vi "GoToPosition.vi"(8 "error in (no error)":errorcluster, 10 "Position":dbl[](array[numeric]), 11 "Serial Controller in":refnum<class "Serial Controller.lvclass">) -> (0 "error out":errorcluster, 3 "Serial Controller out":refnum<class "Serial Controller.lvclass">)   [LabVIEW 2012, in "Serial Controller.lvclass"]
uses:
  Serial Controller.lvclass
  Serial Controller.lvclass/Serial Controller.ctl
panel:
  out "Moving":bool
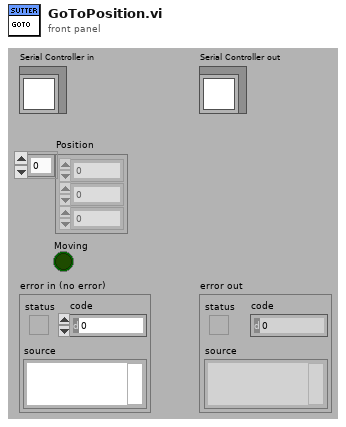
[diagram p1: front panel]
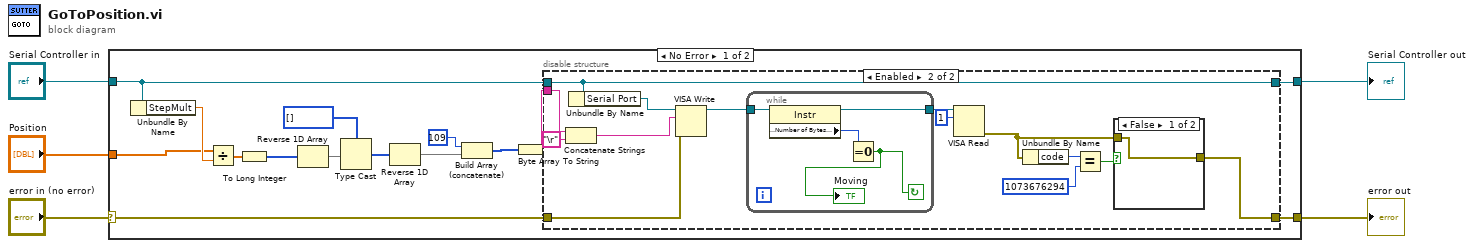
[diagram p0: block diagram]
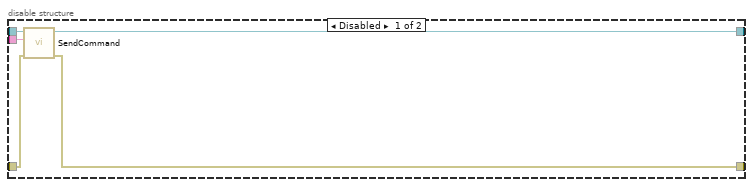
[diagram p2: hidden frame]
diagram:
  n1 = case shown="No Error" "error in (no error)" {
    selector: "error in (no error)" -> [w12 w46]
    tunnel: [w6 w46] -> w4
    tunnel: [w13 w45] -> w2
    tunnel: "Serial Controller in" -> [w14 w45]
    tunnel: "Position" -> [w15 _]
    frame No Error {
      n2 = Unbundle By Name(w14) -> ("StepMult"=w17:dbl)
      n3 = Divide(x=w15, y=w17) -> (x/y=w16:dbl[])
      n4 = To Long Integer(number=w16) -> (32bit integer=w8:i32[])
      n5 = Reverse 1D Array(array=w8) -> (reversed array=w11:i32[])
      n6 = Type Cast(type=u8[] [], x=w11) -> (*(type *) &x=w10:u8[])
      n7 = Reverse 1D Array(array=w10) -> (reversed array=w9:u8[])
      n8 = Build Array (concatenate)(u8 109, w9) -> (w18:u8[])
      n9 = Byte Array To String(unsigned byte array=w18) -> (string=w7:string)
      n10 = disable-structure shown="Enabled" {
        disable-tunnel: w14 -> [w25 w39]
        disable-tunnel: w7 -> [w24 w38]
        disable-tunnel: [w23 w39] -> w13
        disable-tunnel: w12 -> [w21 w34]
        disable-tunnel: [w22 w26] -> w6
        frame Disabled {
          n11 = call-dynamic "SendCommand.vi"("error in (no error)"=w21, "command"=w24, "Serial Controller in"=w25) -> ("error out"=w22:errorcluster, "Serial Controller out"=w23:refnum<class "Serial Controller.lvclass">)  [unwired: 6 in, 1 out]
        }
        frame Enabled {
          n12 = Concatenate Strings(w38, "\r" ("string")) -> (w35:string)
          n13 = Unbundle By Name(w39) -> ("Serial Port"=w36:refnum<visa-resource-name>)
          n14 = VISA Write(VISA resource name=w36, write buffer=w35, error in (no error)=w34) -> (VISA resource name out=w33:refnum<visa-resource-name>)  [unwired: 2 out]
          n15 = while {
            tunnel: w33 -> [w44]
            tunnel: [w42] -> w32
            stop <- w41 continue-if-true
            n16 = property class="Instr"(reference=w44) -> (reference out=w42:refnum<visa-resource-name>, "Serial Settings:Number of Bytes at Serial Port"=w43:u32)  [unwired: 1 in, 1 out]
            n17 = Equal To 0?(x=w43) -> (x = 0?=w41:bool)
            "Moving" <- w41
          }
          n18 = VISA Read(VISA resource name=w32, byte count=u32 1) -> (error out=w27:errorcluster)  [unwired: 1 in, 3 out]
          n19 = Unbundle By Name(w27) -> ("code"=w30:i32)
          n20 = Equal?(x=w30, y=1073676294) -> (x = y?=w28:bool)
          n21 = case shown="False" w28 {
            tunnel: w27 -> [w40 _]
            tunnel: [w40 _] -> w26
            frame False {
            }
            frame True {
            }
          }
        }
      }
    }
    frame Error {
    }
  }
  "error out" <- w4
  "Serial Controller out" <- w2
